vi "Do.vi"(8 "error in":errorcluster, 10 "Actor in":refnum<class "Actor.lvclass">, 11 "Update TE Tech PID":refnum<class "Update TEC PID.lvclass">) -> (0 "error out":errorcluster, 2 "Actor out":refnum<class "Actor.lvclass">)   [LabVIEW 2014, in "Controller.lvlib" / "Update TEC PID.lvclass"]
doc: "(<B>Filename</B>: Actor Framework.lvlib:Message.lvclass:Do.vi)\n\nDefines what a message does when it is received by an actor. Generally, a message instructs an actor to invoke one of its methods. By default, this method does nothing. A child class must override it to define behavior. Create a child class by using the Actor Framework Message Maker dialog box."
uses:
  Update TEC PID.lvclass
  <vilib>/ActorFramework/Actor/Actor.lvclass
  Update TEC PID.lvclass/Update TEC PID.ctl
  Controller.lvclass
  Controls/eMap.ctl
  <vilib>/ActorFramework/Message Enqueuer/Message Enqueuer.lvclass
  Controller.lvclass/Controller.ctl
  SuperActor/SuperActor.lvclass/SuperActor.ctl
  Update TEC PID/Update TEC PID.lvclass
  Update TEC PID/Update TEC PID.lvclass/Update TEC PID.ctl
  <vilib>/ActorFramework/Message Enqueuer/Message Enqueuer.lvclass/Message Enqueuer.ctl
  Update TEC PID/Write ctl.vi
  Accessors/Read Enqueuer Map.vi
  SuperActor/Read Log Session.vi
  <vilib>/ActorFramework/Message Priority Queue/Priority Enqueue.vi
  <userlib>/_Session Fwk/Session - Root.lvclass
  reusable/Session APIs/Session Log/System Log.lvclass
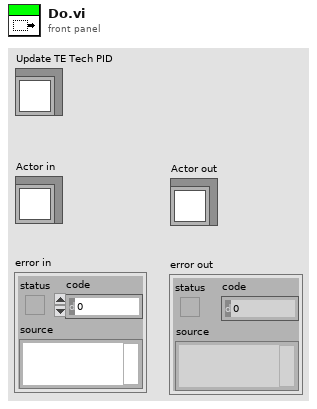
[diagram p1: front panel]
types:
  T1 = typedef "Controller.lvlib/Controller.lvclass/eMap.ctl" = cluster{"Enqueuer":refnum<class "Message Enqueuer.lvclass">, "Active":bool}
  T2 = typedef "Session - Root.lvclass/Session Handle.ctl" = refnum<data-value>
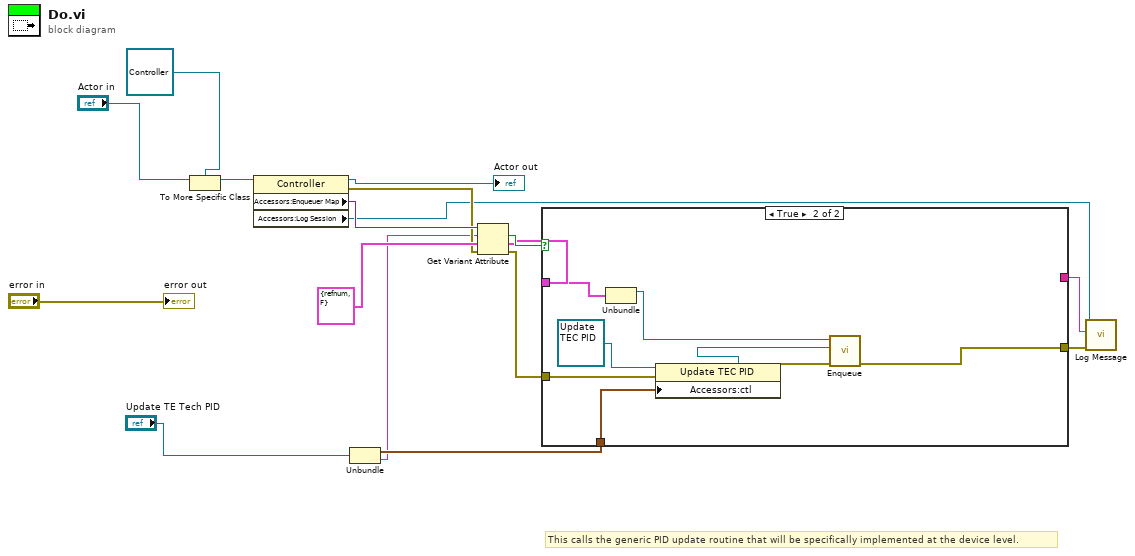
[diagram p0: block diagram]
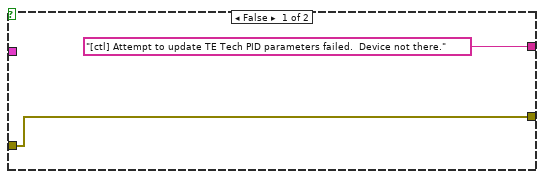
[diagram p2: hidden frame]
diagram:
  # "This calls the generic PID update routine that will be specifically implemented at the device level."
  n1 = To More Specific Class(target class=refnum<class "Controller.lvclass"> refnum ("Controller:Controller"), reference="Actor in") -> (specific class reference=w14:refnum<class "Controller.lvclass">)  [unwired: 1 in, 1 out]
  n2 = property class="Controller"(reference=w14) -> (reference out=→"Actor out":refnum<class "Controller.lvclass">, error out=w7:errorcluster, "Accessors:Enqueuer Map"=w13:variant, "Accessors:Log Session"=w3:T2)  [unwired: 1 in]
  n3 = Unbundle("Update TE Tech PID") -> (w8:cluster{"P":dbl, "I":dbl, "D":dbl}, w1:string)
  n4 = Get Variant Attribute(Variant=w13, name=w1, default value (empty Variant)=T1 {"Enqueuer"=refnum, "Active"=FALSE} ("eMap"), error in=w7) -> (found=w11:bool, value=w10:T1, error out=w6:errorcluster)  [unwired: 1 out]
  n5 = case shown="True" w11 {
    tunnel: w10 -> [_ w27]
    tunnel: w8 -> [_ w24]
    tunnel: w6 -> [w18 w22]
    tunnel: [w18 w20] -> w5
    tunnel: ["[ctl] Attempt to update TE Tech PID parameters failed.  Device not there." _] -> w4
    frame False {
    }
    frame True {
      n6 = Unbundle(w27) -> ("Enqueuer"=w26:refnum<class "Message Enqueuer.lvclass">)  [unwired: 1 out]
      n7 = property class="Update TEC PID"(reference=refnum<class "Update TEC PID.lvclass"> refnum ("TE Cooler.lvlib:Update TEC PID"), error in=w22, "Accessors:ctl"=w24) -> (reference out=w23:refnum<class "Update TEC PID.lvclass">, error out=w21:errorcluster)
      n8 = call <vilib>:"Enqueue.vi"("error in (no error)"=w21, "Message"=w23, "Message Enqueuer in"=w26) -> ("error out"=w20:errorcluster)  [unwired: 7 in, 1 out]
    }
  }
  n9 = call "Log Message.vi"("error in"=w5, "MSG In"=w4, "session in"=w3) -> ()  [unwired: 7 in, 2 out]
  "error out" <- "error in"
